vi "Mouse Overlay.vi"(6 "Event Occured?":bool, 7 "Array In":cluster{"X":i32, "Y":i32}[](array[cluster]), 8 "error in":errorcluster, 9 "Temp Array":dbl[][](array[numeric]), 10 "Last Mouse Position:All Elements":cluster{"X":i32, "Y":i32}, 11 "Image In":T1) -> (0 "error out":errorcluster, 2 "Array Out":cluster{"X":i32, "Y":i32}[](array[cluster]), 3 "Image Out":T1)   [LabVIEW 2023]
doc: "Overlays the Temperature of the last five mouse clicks to the Image Indicator."
uses:
  <vilib>/vision/Image Controls.llb/IMAQ Image.ctl
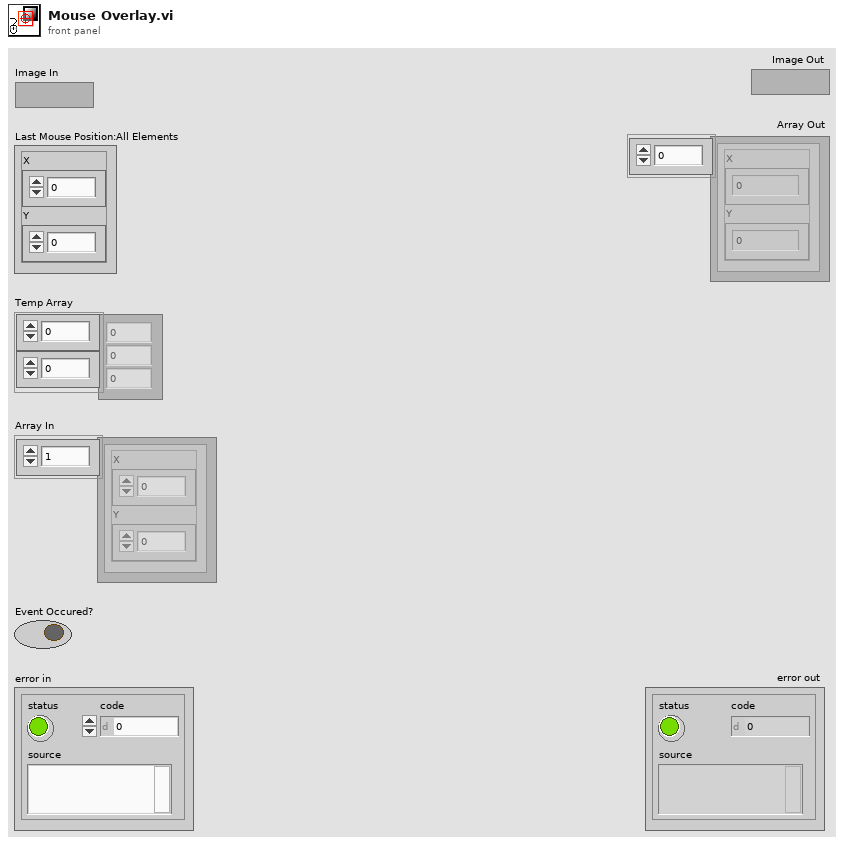
[diagram p1: front panel]
types:
  T1 = typedef "IMAQ Image.ctl" = refnum<image>
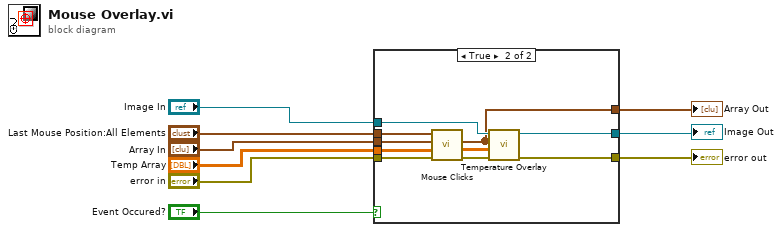
[diagram p0: block diagram]
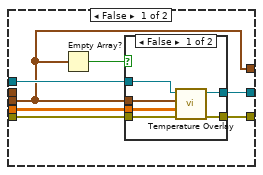
[diagram p2: hidden frame]
diagram:
  n1 = case shown="True" "Event Occured?" {
    tunnel: "error in" -> [w13 w33]
    tunnel: "Image In" -> [w16 w32]
    tunnel: "Temp Array" -> [w14 w30]
    tunnel: [w15 w29] -> w4
    tunnel: [w12 w28] -> w3
    tunnel: [w10 w27] -> w5
    tunnel: "Array In" -> [w10 w26]
    tunnel: "Last Mouse Position:All Elements" -> [_ w25]
    frame False {
      n2 = Empty Array?(array=w10) -> (empty?=w11:bool)
      n3 = case shown="False" w11 {
        tunnel: w16 -> [w22 w23]
        tunnel: [w21 w23] -> w15
        tunnel: w14 -> [w20 _]
        tunnel: w13 -> [w19 w24]
        tunnel: [w18 w24] -> w12
        tunnel: w10 -> [w17 _]
        frame False {
          n4 = call "Temperature Overlay.vi"("error in (no error)"=w19, "Temp Array"=w20, "Array In"=w17, "Image"=w22) -> ("error out"=w18:errorcluster, "Image Out"=w21:T1)  [unwired: 6 in]
        }
        frame True {
        }
      }
    }
    frame True {
      n5 = call "Mouse Clicks.vi"("error in"=w33, "Array In"=w26, "Last Mouse Position:All Elements"=w25) -> ("error out"=w31:errorcluster, "Array Out"=w27:cluster{"X":i32, "Y":i32}[])  [unwired: 7 in]
      n6 = call "Temperature Overlay.vi"("error in (no error)"=w31, "Temp Array"=w30, "Array In"=w27, "Image"=w32) -> ("error out"=w28:errorcluster, "Image Out"=w29:T1)  [unwired: 6 in]
    }
  }
  "Array Out" <- w5
  "Image Out" <- w4
  "error out" <- w3
